vi "Base Empty Only Sub.vi"(8 "P2 disp speed":dbl=5.0, 10 "NaOH steps":u32=500, 11 "FPGA ref in":T1) -> ()   [LabVIEW 2013]
uses:
  Types Def/FPGA Reference.ctl
  <vilib>/rvi/interface/common/niFpgaWaitOnOcc.vi
  <vilib>/Utility/error.llb/Error Cluster From Error Code.vi
  <vilib>/rvi/errors/niLvFpgaAdjustHostInterfaceError.vi
  <vilib>/rvi/interface/nirviReadWriteControl/nirviReadWriteControl.xnode
  NiFpgaLv.dll
  <vilib>/rvi/interface/Simulation/niFpgaSimulationCallBeginRW.vi
panel:
  out "FPGA ref out":T1
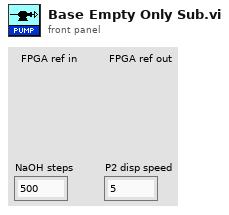
[diagram p1: front panel]
types:
  T1 = typedef "FPGA Reference.ctl" = refnum<k20>
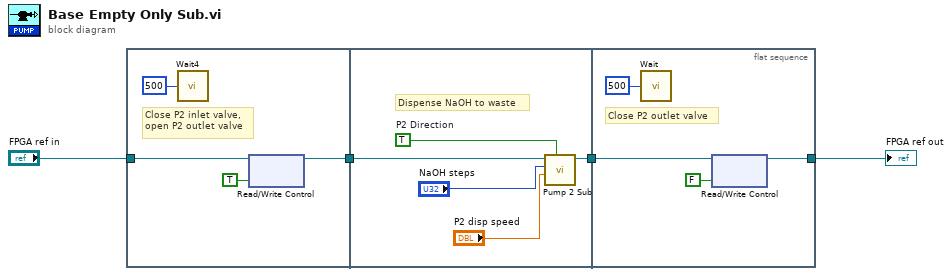
[diagram p0: block diagram]
diagram:
  n1 = flat-sequence {
    tunnel: [w6] -> w4
    tunnel: "FPGA ref in" -> [w5]
    tunnel: w4 -> [w10]
    tunnel: [w12] -> w3
    tunnel: [w16] -> w2
    tunnel: w3 -> [w17]
    frame #0 {
      # "Close P2 inlet valve, \nopen P2 outlet valve"
      n2 = call "Wait4"("Count(mSec)"=u32 500) -> ()  [unwired: 1 out]
      n3 = xnode "Read/Write Control"("FPGA VI Reference In"=w5, "VBDisp"=TRUE ("V2-P1 Waste")) -> ("FPGA VI Reference Out"=w6:T1)  [unwired: 1 in, 1 out]
    }
    frame #1 {
      w13 = TRUE  # P2 Direction
      # "Dispense NaOH to waste"
      n4 = call "Pump 2 Sub.vi"("P2 Direction"=w13, "P2 pps"="P2 disp speed", "P2 Steps"="NaOH steps", "FPGA ref in"=w10) -> ("FPGA ref out"=w12:T1)  [unwired: 6 in, 1 out]
    }
    frame #2 {
      # "Close P2 outlet valve"
      n5 = call "Wait"("Count(mSec)"=u32 500) -> ()  [unwired: 1 out]
      n6 = xnode "Read/Write Control"("FPGA VI Reference In"=w17, "VBDisp"=FALSE ("V4-P2 Waste")) -> ("FPGA VI Reference Out"=w16:T1)  [unwired: 1 in, 1 out]
    }
  }
  "FPGA ref out" <- w2
